vi "Cluster.vi"(8 "error in (no error)":errorcluster, 11 "Node in":refnum<class "Node Config.lvclass">) -> (0 "error out":errorcluster, 2 "Cluster":refnum<class "Cluster Config.lvclass">, 3 "Node out":refnum<class "Node Config.lvclass">)   [LabVIEW 2020, in "VolatusConfig.lvlib" / "Node Config.lvclass"]
uses:
  Node Config.lvclass
  C:/dev/lv20CE/relink/lv-volatus/VolatusConfig/VolatusConfigElement/VolatusConfigElement.lvclass
  Cluster/Cluster Config.lvclass
  Meta Type.ctl
  VolatusConfigElement/VolatusConfigElement.lvclass/VolatusConfigElement.ctl
  VolatusConfigElement/Element.vi
  lv-cdm/CDM-Config/Config Lookup/Match Meta.vi
  lv-cdm/CDM-Config/Config Element/Owner.vi
  lv-cdm/CDM-Config/Config Filter/Config Lookup.lvclass
  Node Config.lvclass/Node Config.ctl
  VolatusConfigElement/VolatusConfigElement.lvclass
  VolatusConfig.lvlib
  C:/dev/lv20CE/relink/lv-volatus/VolatusConfig/Node/Node Config.lvclass
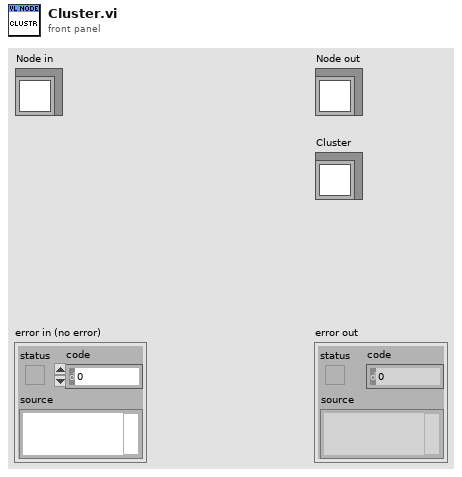
[diagram p1: front panel]
types:
  T1 = typedef "VolatusConfig.lvlib/Meta Type.ctl" = enum16{"UNKNOWN", "VL_System", "VL_Cluster", "VL_Node", "VL_Task", "VL_Group", "VL_Channel", "VL_Task_List", "VL_Scaling", "VL_Sensor", "VL_Sensor_List", "VL_Scale"}
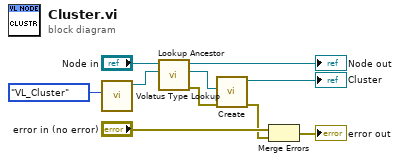
[diagram p0: block diagram]
diagram:
  n1 = call "Volatus Type Lookup.vi"("Meta Type"=Meta_Type."VL_Cluster") -> ("Config Lookup out"=w7:refnum<class "Config Lookup.lvclass">)  [unwired: 9 in, 1 out]
  n2 = call "Lookup Ancestor.vi"("Lookup"=w7, "VolatusConfigElement in"="Node in") -> ("error out"=w5:errorcluster, "Ancestor"=w6:refnum<class "Config Element.lvclass">, "VolatusConfigElement out"=→"Node out":refnum<class "Node Config.lvclass">)  [unwired: 7 in]
  n3 = call "Create.vi"("error in (no error)"=w5, "Element"=w6) -> ("error out"=w2:errorcluster, "Cluster out"=→"Cluster":refnum<class "Cluster Config.lvclass">)  [unwired: 8 in]
  n4 = Merge Errors("error in (no error)", w2) -> (→"error out":errorcluster)
